vi "TestInitializeBasicPolicy_PublishOK.vi"(8 "error in (no error)":errorcluster, 11 "TestCase in":refnum<class "TestSubscriptionPolicy.lvclass">) -> (0 "error out":errorcluster, 3 "TestCase out":refnum<class "TestSubscriptionPolicy.lvclass">)   [LabVIEW 2020, in "TestSubscriptionPolicy.lvclass"]
uses:
  TestSubscriptionPolicy.lvclass
  TestSubscriptionPolicy.lvclass/TestSubscriptionPolicy.ctl
  Source/IMediator/ISubscriptionPolicy/ISubscriptionPolicy.lvclass
  Source/SubscriptionPolicy/BasicSubscription/BasicSubscription.lvclass
  modules/composed-transport/Source/Concrete/QueueTransport/QueueTransport.lvclass
  C:/Git/mva-core/Source/IMediator/ISubscriptionPolicy/ISubscriptionPolicy.lvclass
  C:/Git/mva-core/Source/SubscriptionPolicy/BasicSubscription/BasicSubscription.lvclass
  C:/Git/mva-core/modules/composed-transport/Source/ITransport/ITransport.lvclass
  C:/Git/mva-core/modules/composed-transport/Source/Concrete/QueueTransport/QueueTransport.lvclass
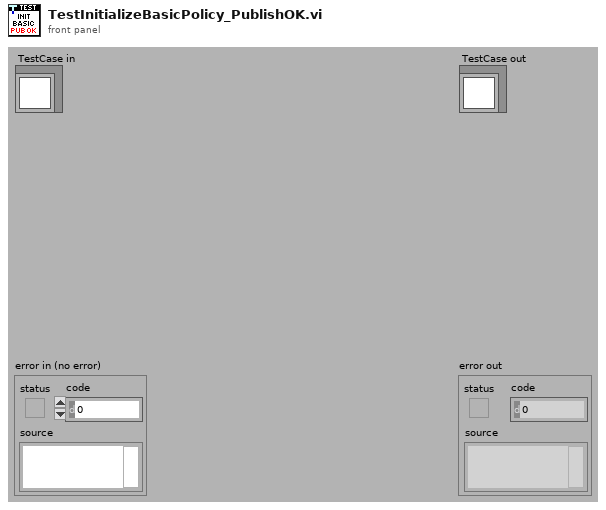
[diagram p1: front panel]
types:
  T1 = typedef "IMediator.lvlib/ISubscriptionPolicy.lvclass/ISubscriptionPolicy Reference.ctl" = refnum<data-value>
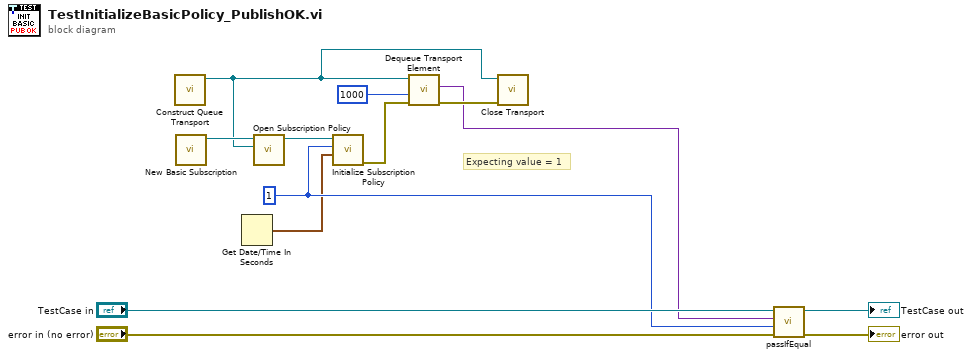
[diagram p0: block diagram]
diagram:
  w6 = 1
  # "Expecting value = 1"
  n1 = call "Construct Queue Transport.vi"() -> ("QueueTransport"=w1:refnum<class "QueueTransport.lvclass">)  [unwired: 10 in, 1 out]
  n2 = call "New Basic Subscription.vi"() -> ("BasicSubscription Out"=w3:refnum<class "BasicSubscription.lvclass">)  [unwired: 11 in]
  n3 = Get Date/Time In Seconds() -> (seconds since 1Jan1904=w5:timestamp)
  n4 = call "Open Subscription Policy.vi"("Transport"=w1, "SubscriptionPolicy"=w3) -> ("Subscription Policy"=w9:T1)  [unwired: 8 in, 1 out]
  n5 = call "Initialize Subscription Policy.vi"("Last Publish Time"=w5, "Last Topic Value"=w6, "Subscription Policy"=w9) -> ("Error Out (Unsubscribe?)"=w8:errorcluster)  [unwired: 7 in, 1 out]
  n6 = call "Dequeue Transport Element.vi"("error in (no error)"=w8, "Timeout In ms (-1)"=1000, "QueueTransport"=w1) -> ("error out"=w4:errorcluster, "Data"=w2:variant)  [unwired: 5 in, 2 out]
  n7 = call-dynamic "Close Transport.vi"("error in (no error)"=w4, "QueueTransport"=w1) -> ()  [unwired: 9 in, 1 out]
  n8 = call-dynamic "passIfEqual.vi"("error in (no error)"="error in (no error)", "y"=w6, "x"=w2, "TestCase in"="TestCase in") -> ("error out"=→"error out":errorcluster, "TestCase out"=→"TestCase out":refnum<class "TestSubscriptionPolicy.lvclass">)  [unwired: 6 in]
